vi "Abort Single Point-Ganging.vi"(8 "error in":errorcluster, 11 "Ganged Session Out":T1) -> (0 "error out":errorcluster)   [LabVIEW 2021]
doc: "Abort the single point. In case of error resets the device for ganging configuration."
uses:
  controls/Abort Single Point-Ganging.ctl
  channel ganging/shared subVIs/ctl/NIDCPower_channel_ganging - ctl - ganged config.ctl
  channel ganging/shared subVIs/ctl/NIDCPower_channel_ganging - ctl - channel mode.ctl
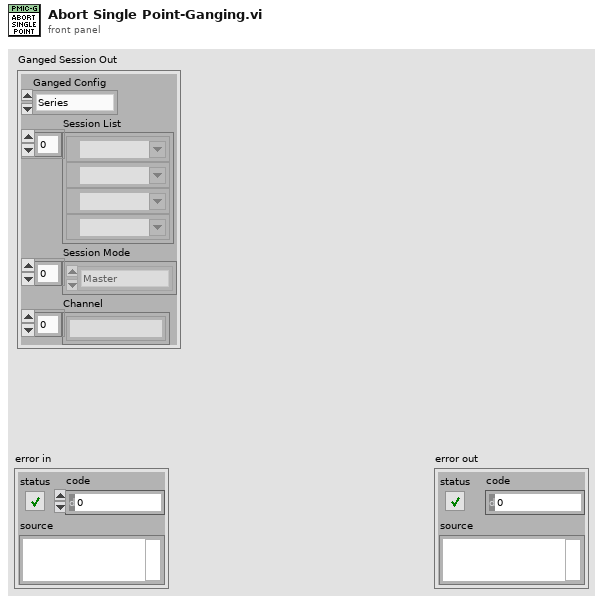
[diagram p1: front panel]
types:
  T1 = typedef "Abort Single Point-Ganging.ctl" = cluster{"Ganged Config":T2, "Session List":refnum<k15>[], "Session Mode":T3[], "Channel":string[]}
  T2 = typedef "NIDCPower_channel_ganging - ctl - ganged config.ctl" = enum32{"Series", "Parallel", "Manual"}
  T3 = typedef "NIDCPower_channel_ganging - ctl - channel mode.ctl" = enum32{"Master", "Slave", "Slave - Inverted"}
  T4 = typedef "NIDCPower_channel_ganging - ctl - ganged session.ctl" = cluster{"Ganged Config":T2, "Session List":refnum<k15>[], "Session Mode":T3[], "Channel":string[]}
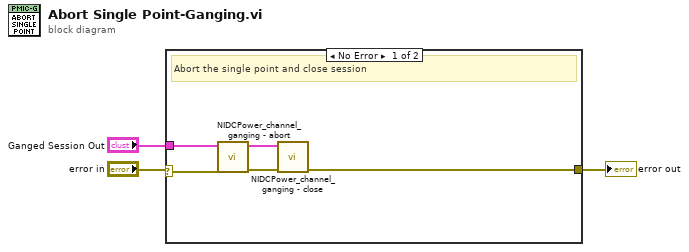
[diagram p0: block diagram]
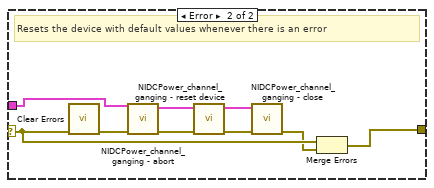
[diagram p2: hidden frame]
diagram:
  n1 = case shown="No Error" "error in" {
    selector: "error in" -> [w8 w11]
    tunnel: "Ganged Session Out" -> [w4 w13]
    tunnel: [w7 w9] -> w2
    frame No Error {
      # "Abort the single point and close session"
      n2 = call "NIDCPower_channel_ganging - abort.vi"("error in (no error)"=w8, "Ganged Session In"=w4) -> ("error out"=w5:errorcluster, "Ganged Session Out"=w6:T4)  [unwired: 8 in]
      n3 = call "NIDCPower_channel_ganging - close.vi"("error in (no error)"=w5, "Ganged Session In"=w6) -> ("error out"=w7:errorcluster)  [unwired: 9 in]
    }
    frame Error {
      # "Resets the device with default values whenever there is an error"
      n4 = call <vilib>:"Clear Errors.vi"("error in (no error)"=w11) -> ("error out"=w12:errorcluster)  [unwired: 5 in, 1 out]
      n5 = call "NIDCPower_channel_ganging - abort.vi"("error in (no error)"=w12, "Ganged Session In"=w13) -> ("error out"=w16:errorcluster, "Ganged Session Out"=w17:T4)  [unwired: 8 in]
      n6 = call "NIDCPower_channel_ganging - reset device.vi"("error in (no error)"=w16, "Ganged Session In"=w17) -> ("error out"=w14:errorcluster, "Ganged Session Out"=w15:T4)  [unwired: 8 in]
      n7 = call "NIDCPower_channel_ganging - close.vi"("error in (no error)"=w14, "Ganged Session In"=w15) -> ("error out"=w10:errorcluster)  [unwired: 9 in]
      n8 = Merge Errors(w11, w10) -> (w9:errorcluster)
    }
  }
  "error out" <- w2
